vi "ATE_Panel.vi"() -> ()   [LabVIEW 2009]
panel:
  out "error out":errorcluster
  in  "TimeOut":i32
  in  "Amp32dB":bool
  out "121 dB attn":bool[](array[boolean])=[FALSE, TRUE, TRUE, TRUE, TRUE, TRUE, TRUE, TRUE, TRUE]
  out "70 dB attn":bool[](array[boolean])=[FALSE, TRUE, TRUE, TRUE]
  in  "stop":bool
  in  "121 dB":bool
  in  "70 dB":bool
  in  "70 dB Attn":i32=70 min=0 max=70 step=10
  in  "121 dB Attn":i32=121 min=0 max=121 step=1
  # "32 dB Amp"
  # "1 dB"
  # "2 dB"
  # "4 dB"
  # "4 dB"
  # "10 dB"
  # "20 dB"
  # "40 dB"
  # "40 dB"
  # "10 dB"
  # "20 dB"
  # "40 dB"
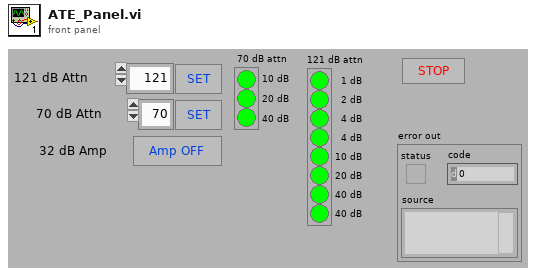
[diagram p1: front panel]
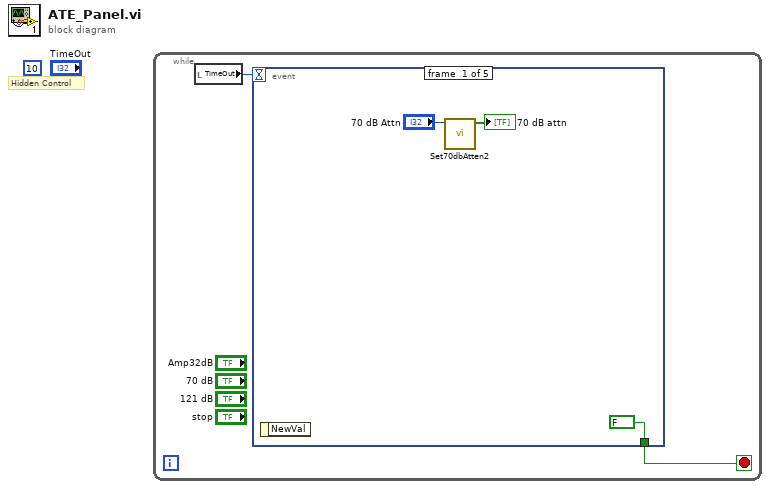
[diagram p0: block diagram]
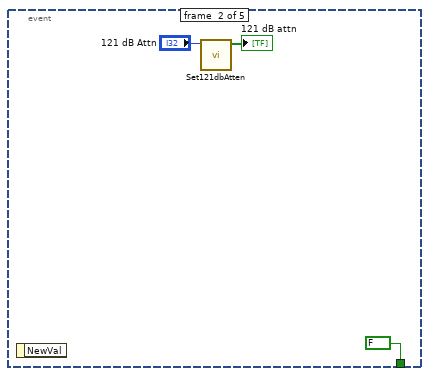
[diagram p2: hidden frame]
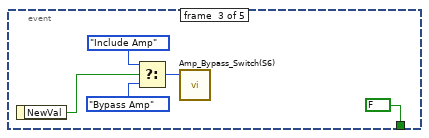
[diagram p3: hidden frame]
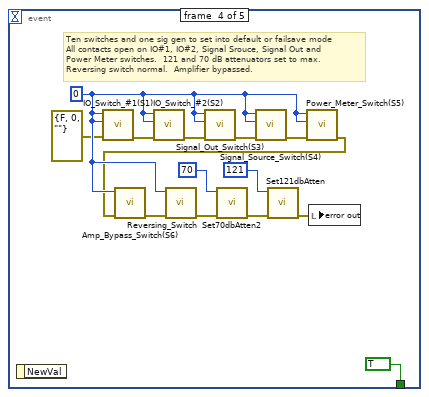
[diagram p4: hidden frame]
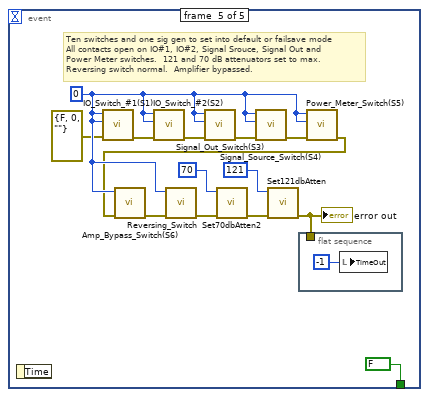
[diagram p5: hidden frame]
diagram:
  (unwired) 10 ("TimeOut")
  # "Hidden Control"
  n1 = while {
    stop <- w2 stop-if-true
    n2 = local read "TimeOut"() -> (w1:i32)
    n3 = event shown="[4] Timeout" {
      selector: _ -> [_ _ _ _ _]
      dyn-events: _ -> [_ _ _ _ _]
      timeout: w1 -> [_ _ _ _ _]
      tunnel: [FALSE ("NewVal") FALSE ("NewVal") FALSE ("NewVal") TRUE ("NewVal") FALSE ("NewVal")] -> w2
      event #0 {
        n4 = event-data() -> ()  [unwired: 1 in, 1 out]
        n5 = call "Set70dbAtten2.vi"("Attenuation (dB)"="70 dB Attn") -> ("Active Attenuators"=→"70 dB attn":bool[])  [unwired: 9 in, 1 out]
      }
      event #1 {
        n6 = event-data() -> ()  [unwired: 1 in, 1 out]
        n7 = call "Set121dbAtten.vi"("Attenuation (dB)"="121 dB Attn") -> ("Active Attenuators"=→"121 dB attn":bool[])  [unwired: 9 in, 1 out]
      }
      event #2 {
        n8 = event-data() -> ("NewVal"=w13:bool)  [unwired: 1 in]
        n9 = Select(t=enum16{"Bypass Amp", "Include Amp"}."Include Amp" ("AMP Function"), s=w13, f=enum16{"Bypass Amp", "Include Amp"}."Bypass Amp" ("AMP Function")) -> (s? t:f=w10:enum16{"Bypass Amp", "Include Amp"})
        n10 = call "Amp_Bypass_Switch(S6).vi"("AMP Function"=w10) -> ()  [unwired: 10 in, 1 out]
      }
      event #3 {
        w26 = u16 0
        # "Ten switches and one sig gen to set into default or failsave mode\nAll contacts open on IO#1, IO#2, Signal Srouce, Signal Out and \nPower Meter switches.  121 and 70 dB attenuators set to max.\nReversing switch normal.  Amplifier bypassed."
        n11 = event-data() -> ()  [unwired: 1 in, 1 out]
        n12 = call "IO_Switch_#1(S1).vi"("error in"=errorcluster {"status"=FALSE, "code"=0, "source"=""}, "Output"=w26, "Input"=w26) -> ("error out"=w22:errorcluster)  [unwired: 7 in, 1 out]
        n13 = call "IO_Switch_#2(S2).vi"("error in"=w22, "Output"=w26, "Input"=w26) -> ("error out"=w21:errorcluster)  [unwired: 7 in, 1 out]
        n14 = call "Signal_Out_Switch(S3).vi"("error in"=w21, "Output"=w26, "Input"=w26) -> ("error out"=w20:errorcluster)  [unwired: 7 in, 1 out]
        n15 = call "Signal_Source_Switch(S4).vi"("error in"=w20, "Output"=w26, "Input"=w26) -> ("error out"=w19:errorcluster)  [unwired: 7 in, 1 out]
        n16 = call "Power_Meter_Switch(S5).vi"("error in"=w19, "Output"=w26, "Input"=w26) -> ("error out"=w18:errorcluster)  [unwired: 7 in, 1 out]
        n17 = call "Amp_Bypass_Switch(S6).vi"("error in"=w18, "AMP Function"=w26) -> ("error out"=w17:errorcluster)  [unwired: 9 in]
        n18 = call "Reversing_Switch.vi"("error in"=w17, "Reversing Switch Function"=w26) -> ("error out"=w16:errorcluster)  [unwired: 9 in]
        n19 = call "Set70dbAtten2.vi"("error in (no error)"=w16, "Attenuation (dB)"=70) -> ("error out"=w15:errorcluster)  [unwired: 8 in, 1 out]
        n20 = call "Set121dbAtten.vi"("error in (no error)"=w15, "Attenuation (dB)"=121) -> ("error out"=w14:errorcluster)  [unwired: 8 in, 1 out]
        n21 = local write "error out"(w14) -> ()
      }
      event #4 {
        w40 = u16 0
        # "Ten switches and one sig gen to set into default or failsave mode\nAll contacts open on IO#1, IO#2, Signal Srouce, Signal Out and \nPower Meter switches.  121 and 70 dB attenuators set to max.\nReversing switch normal.  Amplifier bypassed."
        n22 = event-data() -> ()  [unwired: 1 in, 1 out]
        n23 = call "IO_Switch_#1(S1).vi"("error in"=errorcluster {"status"=FALSE, "code"=0, "source"=""}, "Output"=w40, "Input"=w40) -> ("error out"=w36:errorcluster)  [unwired: 7 in, 1 out]
        n24 = call "IO_Switch_#2(S2).vi"("error in"=w36, "Output"=w40, "Input"=w40) -> ("error out"=w35:errorcluster)  [unwired: 7 in, 1 out]
        n25 = call "Signal_Out_Switch(S3).vi"("error in"=w35, "Output"=w40, "Input"=w40) -> ("error out"=w34:errorcluster)  [unwired: 7 in, 1 out]
        n26 = call "Signal_Source_Switch(S4).vi"("error in"=w34, "Output"=w40, "Input"=w40) -> ("error out"=w33:errorcluster)  [unwired: 7 in, 1 out]
        n27 = flat-sequence {
          tunnel: w28 -> [_]
          frame #0 {
            n28 = local write "TimeOut"(-1 ("TimeOut")) -> ()
          }
        }
        n29 = call "Power_Meter_Switch(S5).vi"("error in"=w33, "Output"=w40, "Input"=w40) -> ("error out"=w32:errorcluster)  [unwired: 7 in, 1 out]
        n30 = call "Amp_Bypass_Switch(S6).vi"("error in"=w32, "AMP Function"=w40) -> ("error out"=w31:errorcluster)  [unwired: 9 in]
        n31 = call "Reversing_Switch.vi"("error in"=w31, "Reversing Switch Function"=w40) -> ("error out"=w30:errorcluster)  [unwired: 9 in]
        n32 = call "Set70dbAtten2.vi"("error in (no error)"=w30, "Attenuation (dB)"=70) -> ("error out"=w29:errorcluster)  [unwired: 8 in, 1 out]
        n33 = call "Set121dbAtten.vi"("error in (no error)"=w29, "Attenuation (dB)"=121) -> ("error out"=w28:errorcluster)  [unwired: 8 in, 1 out]
        "error out" <- w28
      }
    }
  }
